vi "XML_getClosingTag.vi"(9 "tag":string, 11 "XML In":string) -> (0 "after tag":string, 1 "closing tag":string, 3 "before tag":string)   [LabVIEW 2012]
uses:
  <vilib>/regexp/Match Regular Expression.xnode
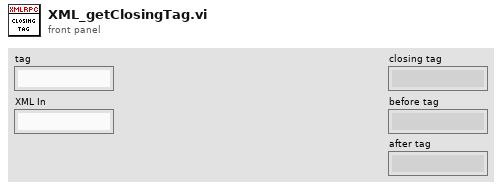
[diagram p1: front panel]
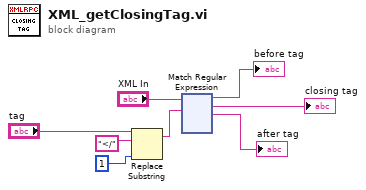
[diagram p0: block diagram]
diagram:
  n1 = Replace Substring(2:1 ("length (len. of substring)"), 4:"</" ("substring (\"\")"), 5:"tag") -> (1:w6:string)  [unwired: 1 in, 1 out]
  n2 = xnode "Match Regular Expression"("input string"="XML In", "regular expression"=w6) -> ("before match"=→"before tag":string, "whole match"=→"closing tag":string, "after match"=→"after tag":string)  [unwired: 4 in, 2 out]
